vi "Initiate.vi"(8 "error in (no error)":errorcluster, 11 "IVI_DMM in":refnum<class "IVI_DMM.lvclass">) -> (0 "error out":errorcluster, 3 "IVI_DMM out":refnum<class "IVI_DMM.lvclass">)   [LabVIEW 2013, in "IVI_DMM.lvlib" / "IVI_DMM.lvclass"]
doc: "This VI initiates a measurement. After you call this VI, the DMM leaves the Idle state and waits for a trigger.\n\nThis VI applies default values to properties that have not been set by the user under the following conditions:\n\n(1) If the user has not set the value of any property in the IviDmmMultiPoint extension group, the VI sets the IviDmm>>Multi-Point Acquisition>>Sample Count [MP] and IviDmm>>Multi-Point Acquisition>>Trigger Count [MP] properties to 1.\n\n(2) If the user has not set the value of the IviDmm>Measurement Operation Options>Auto Zero [AZ] property, the VI sets the value of this property to IVIDMM_VAL_AUTO_ZERO_OFF (0). \n\nNotes:\n\n(1) This VI does not check the instrument status. Typically, you call this VI only in a sequence of calls to other low-level driver VIs. The sequence performs one operation. You use the low-level VIs to optimize one or more aspects of interaction with the instrument. If you want to check the instrument status, call the IviDmm Error-Query VI at the conclusion of the sequence.\n\n(2) This VI performs interchangeability checking when the IviDmm>>Inherent IVI Settings>>User Options>>Interchange Check property is set to TRUE. If the IviDmm>>Inherent IVI Settings>>User Options>>Spy property is set to TRUE, you use the NI I/O Trace utility to view interchangeability warnings. You use the IviDmm Get Next Interchange Warning VI to retrieve interchangeability warnings when the IviDmm>>Inherent IVI Settings>>User Options>>Spy property is set to FALSE. For more information about interchangeability checking, refer to the help text for the IviDmm>>Inherent IVI Settings>>User Options>>Interchange Check property.\n\n(3) The class driver initiates a simulated measurement when this VI is called and the IviDmm>>Inherent IVI Settings>>User Options>>Simulate property is set to TRUE and the IviDmm>>Inherent IVI Settings>>User Options>>Use Specific Simulation property is set to FALSE. For information on how to configure a simulated measurement, refer to the online help manual."
uses:
  IVI_DMM.lvclass
  IVI_DMM.lvclass/IVI_DMM.ctl
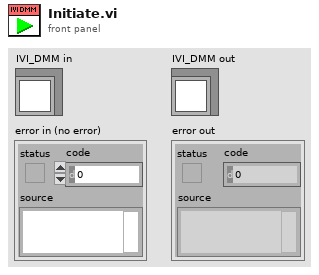
[diagram p1: front panel]
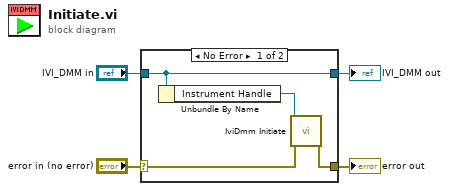
[diagram p0: block diagram]
diagram:
  n1 = case shown="No Error" "error in (no error)" {
    selector: "error in (no error)" -> [w6 w10]
    tunnel: [w5 w10] -> w3
    tunnel: [w8 w9] -> w1
    tunnel: "IVI_DMM in" -> [w8 w9]
    frame No Error {
      n2 = Unbundle By Name(w8) -> ("Instrument Handle"=w7:refnum<k15>)
      n3 = call <vilib>:"IviDmm Initiate.vi"("error in (no error)"=w6, "instrument handle"=w7) -> ("error out"=w5:errorcluster)  [unwired: 8 in, 1 out]
    }
    frame Error {
    }
  }
  "error out" <- w3
  "IVI_DMM out" <- w1
